vi "Rem Write Handshake.vi"(0 "Handshake":bool, 1 "String In":string, 2 "File Path Control":path) -> (10 "error out":errorcluster)   [LabVIEW 2014]
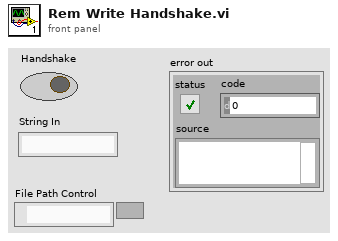
[diagram p1: front panel]
types:
  T1 = enum16{"open", "replace", "create", "open or create", "replace or create", "replace or create with confirmation"}
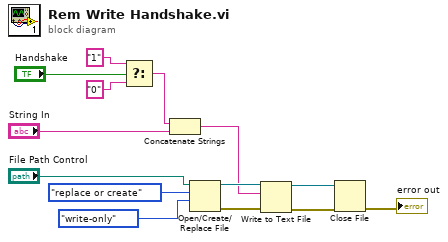
[diagram p0: block diagram]
diagram:
  n1 = Select(t="1" ("text"), s="Handshake", f="0" ("text")) -> (s? t:f=w4:string)
  n2 = Concatenate Strings(w4, "String In") -> (w2:string)
  n3 = Open/Create/Replace File(file path (use dialog)="File Path Control", operation (0:open)=T1."replace or create", access (0:read/write)=enum16{"read/write", "read-only", "write-only"}."write-only") -> (refnum out=w11:refnum<file>, error out=w10:errorcluster)  [unwired: 3 in, 1 out]
  n4 = Write to Text File(file (use dialog)=w11, text=w2, error in=w10) -> (refnum out=w12:refnum<file>, error out=w13:errorcluster)  [unwired: 1 in, 1 out]
  n5 = Close File(refnum=w12, error in=w13) -> (error out=→"error out":errorcluster)  [unwired: 1 out]
